vi "OC_SC_Detection.vi"() -> (2 "Open Loop Channels Array":bool[](array[boolean]), 3 "Short Circuit Channels Array":bool[](array[boolean]))   [LabVIEW 2017, in "BOP_VibAPI_4.lvlib"]
uses:
  <vilib>/addons/InsightCM/Devices/Shared/Cms/Fpga/Acquisition/source/subVIs/VibAPI_4/BOP_VibAPI_4.lvlib
  <vilib>/rvi/eio/common/nirviEmuTemplateMethod_errors.vi
  <vilib>/eio/EIOMethodNode/EIOMethodNode.xnode
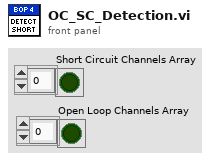
[diagram p1: front panel]
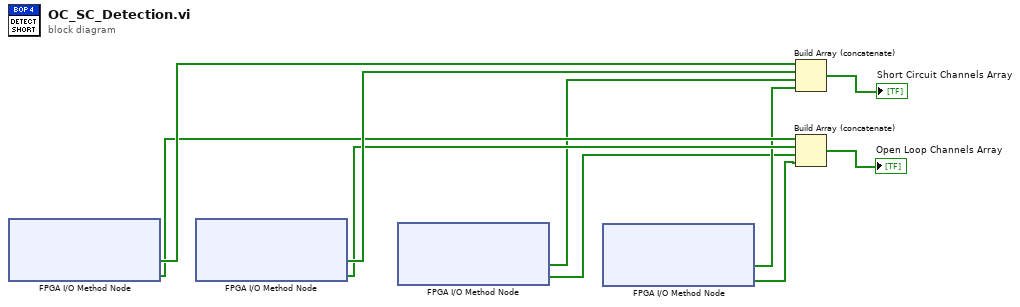
[diagram p0: block diagram]
diagram:
  n1 = xnode "FPGA I/O Method Node"() -> ("Short Circuit"=w10:bool[], "Open Loop"=w8:bool[])  [unwired: 1 in, 1 out]
  n2 = xnode "FPGA I/O Method Node"() -> ("Short Circuit"=w9:bool[], "Open Loop"=w7:bool[])  [unwired: 1 in, 1 out]
  n3 = xnode "FPGA I/O Method Node"() -> ("Short Circuit"=w4:bool[], "Open Loop"=w1:bool[])  [unwired: 1 in, 1 out]
  n4 = xnode "FPGA I/O Method Node"() -> ("Short Circuit"=w3:bool[], "Open Loop"=w2:bool[])  [unwired: 1 in, 1 out]
  n5 = Build Array (concatenate)(w10, w9, w4, w3) -> (→"Short Circuit Channels Array":bool[])
  n6 = Build Array (concatenate)(w8, w7, w1, w2) -> (→"Open Loop Channels Array":bool[])
